vi "subDFD_Show Busy.vi"() -> ()   [LabVIEW 2017]
panel:
  out "String":string="Please wait..."
  in  "exit":bool
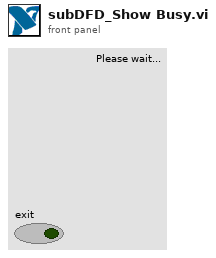
[diagram p1: front panel]
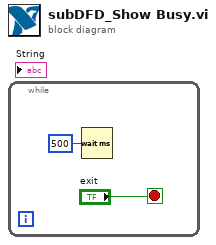
[diagram p0: block diagram]
diagram:
  n1 = while {
    stop <- "exit" stop-if-true
    n2 = Wait (ms)(milliseconds to wait=u32 500) -> ()  [unwired: 1 out]
  }
